vi "Filter_ext.vi"(4 "dT":dbl=1.0 min=1.0 max=3600000.0 format="%#_3g", 6 "PV_OUT old":dbl format="%#_3g", 9 "time_const ms":dbl=1.0 min=1.0 max=3600000.0 format="%#_3g", 10 "PV":dbl format="%#_3g", 11 "Initialise":bool) -> (3 "PV_OUT":dbl format="%#_3g")   [LabVIEW 2019, in "Userlib.lvlib"]
uses:
  Userlib.lvlib
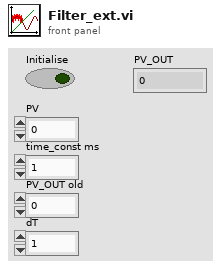
[diagram p1: front panel]
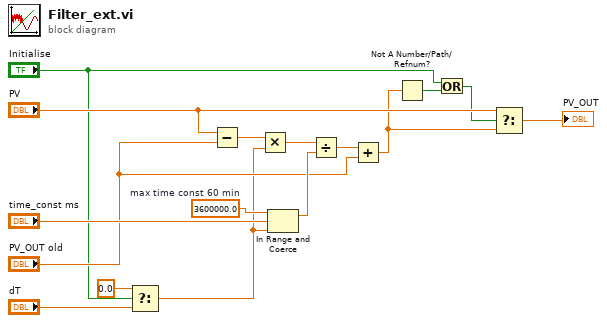
[diagram p0: block diagram]
diagram:
  w12 = 3600000.0  # max time const 60 min
  n1 = Select(t=0.0, s="Initialise", f="dT") -> (s? t:f=w1:dbl)
  n2 = Subtract(x="PV", y="PV_OUT old") -> (x-y=w16:dbl)
  n3 = Multiply(x=w16, y=w1) -> (x*y=w15:dbl)
  n4 = In Range and Coerce(upper limit=w12, x="time_const ms", lower limit=w1) -> (coerced(x)=w14:dbl)  [unwired: 1 out]
  n5 = Divide(x=w15, y=w14) -> (x/y=w11:dbl)
  n6 = Add(x=w11, y="PV_OUT old") -> (x+y=w8:dbl)
  n7 = Not A Number/Path/Refnum?(number/path/refnum=w8) -> (NaN/Path/Refnum?=w7:bool)
  n8 = Or(x="Initialise", y=w7) -> (x .or. y?=w6:bool)
  n9 = Select(t="PV", s=w6, f=w8) -> (s? t:f=→"PV_OUT":dbl)
